vi "TVA_cmd (SubVI).vi"(4 "W_b [rad/s]":dbl[](array[numeric]), 6 "Angles [rad]":dbl[](array[numeric]), 8 "TVA_old [rad]":dbl[](array[numeric]), 11 "TVA_cmd [rad]":dbl[](array[numeric])) -> (2 "Act315_Act225":dbl[](array[numeric]), 3 "TVA_b":dbl[](array[numeric]))   [LabVIEW 2017]
panel:
  out "roll1":dbl
  out "TVA_control_time [s]":dbl
  in  "T [s]":dbl format="%#_13g"
  out "roll_angle [rad]":dbl
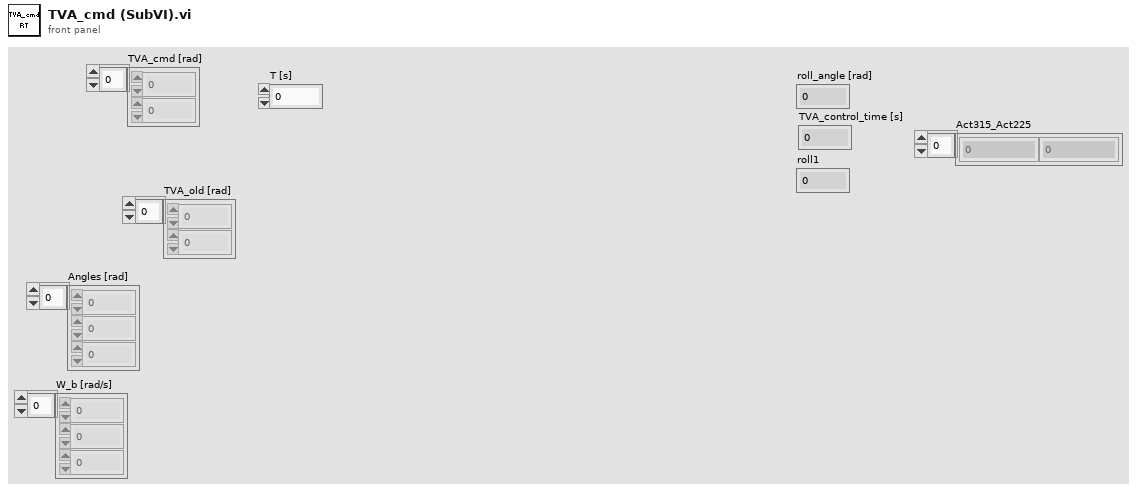
[diagram p1: front panel]
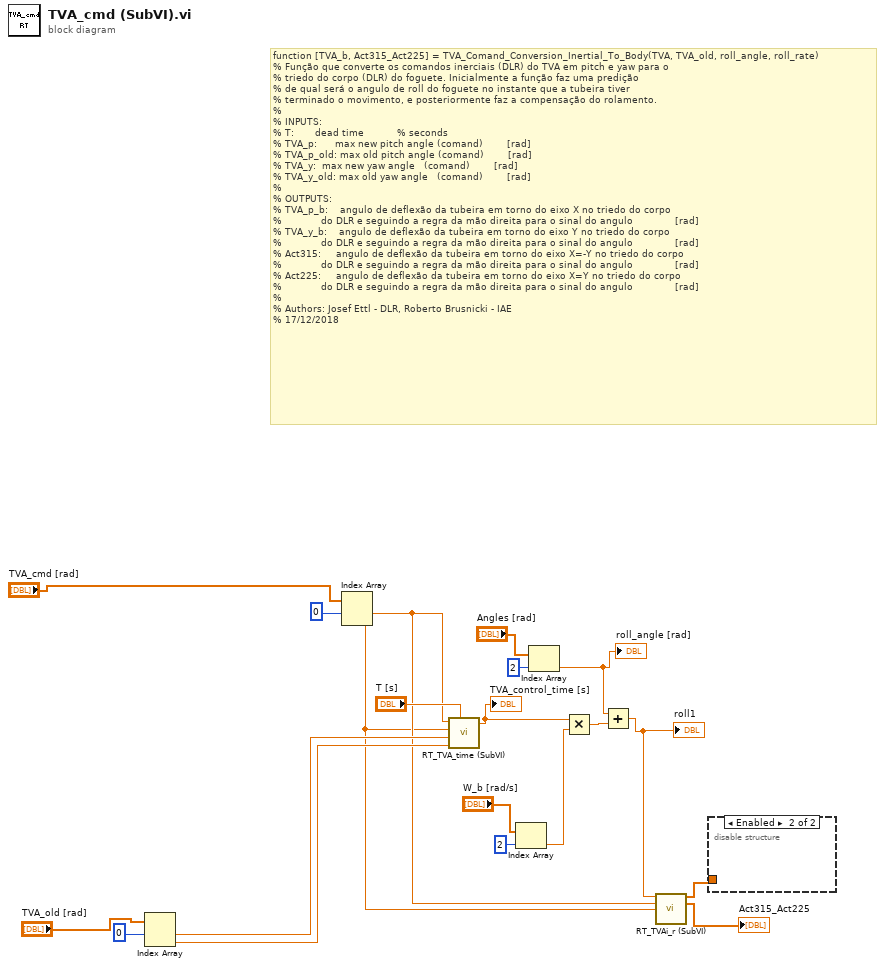
[diagram p0: block diagram]
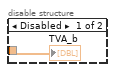
[diagram p2: hidden frame]
diagram:
  # "function [TVA_b, Act315_Act225] = TVA_Comand_Conversion_Inertial_To_Body(TVA, TVA_old, roll_angle, roll_rate)\n% Função que converte os comandos inerciais (DLR) do TVA em pitch e yaw para o\n% triedo do corpo (DLR) do foguete. Inicialmente a função faz uma predição\n% de qual será o angulo de roll do foguete no instante que a tubeira tiver\n% terminado o movimento, e posteriormente faz a compensação do rolamento.\n%\n% INPUTS:\n% T: \t\t    dead time           % seconds  \n% TVA_p: \t    max new pitch angle (comand)        [rad]\n% TVA_p_old:\tmax old pitch angle (comand)        [rad]\n% TVA_y:\t\tmax new yaw angle   (comand)        [rad]\n% TVA_y_old:\tmax old yaw angle   (comand)        [rad]\n%\n% OUTPUTS:\n% TVA_p_b:    angulo de deflexão da tubeira em torno do eixo X no triedo do corpo\n%             do DLR e seguindo a regra da mão direita para o sinal do angulo              [rad]\n% TVA_y_b:    angulo de deflexão da tubeira em torno do eixo Y no triedo do corpo\n%             do DLR e seguindo a regra da mão direita para o sinal do angulo              [rad]\n% Act315:     angulo de deflexão da tubeira em torno do eixo X=-Y no triedo do corpo\n%             do DLR e seguindo a regra da mão direita para o sinal do angulo              [rad]\n% Act225:     angulo de deflexão da tubeira em torno do eixo X=Y no triedo do corpo\n%             do DLR e seguindo a regra da mão direita para o sinal do angulo              [rad]\n% \n% Authors: Josef Ettl - DLR, Roberto Brusnicki - IAE\n% 17/12/2018"
  n1 = Index Array(array="TVA_old [rad]", index #1=0 ("disabled index (col)")) -> (element #1=w16:dbl, element #2=w15:dbl)  [unwired: 1 in]
  n2 = Index Array(array="TVA_cmd [rad]", index #1=0 ("disabled index (col)")) -> (element #1=w14:dbl, element #2=w13:dbl)  [unwired: 1 in]
  n3 = call "RT_TVA_time (SubVI).vi"("T [s]"="T [s]", "TVA_y_old"=w15, "TVA_p_old"=w16, "TVA_y"=w13, "TVA_p"=w14) -> ("TVA_control_time [s]"=w2:dbl)  [unwired: 6 in]
  "TVA_control_time [s]" <- w2
  n4 = Index Array(array="W_b [rad/s]", index=2) -> (element=w3:dbl)
  n5 = Index Array(array="Angles [rad]", index=2) -> (element=w9:dbl)
  "roll_angle [rad]" <- w9
  n6 = Multiply(x=w2, y=w3) -> (x*y=w4:dbl)
  n7 = Add(x=w9, y=w4) -> (x+y=w10:dbl)
  "roll1" <- w10
  n8 = call "RT_TVAi_r (SubVI).vi"("roll1"=w10, "TVA_p"=w14, "TVA_y"=w13) -> ("TVA_b"=w8:dbl[], "Act315_Act225"=→"Act315_Act225":dbl[])  [unwired: 11 in]
  n9 = disable-structure shown="Enabled" {
    disable-tunnel: w8 -> [w21 _]
    frame Disabled {
      "TVA_b" <- w21
    }
    frame Enabled {
    }
  }
